vi "Add Project.vi"(6 "Tasks Active?":bool[](array[boolean]), 7 "Add Default Tasks (T)":bool=TRUE, 8 "error in (no error)":errorcluster, 9 "Tasks":string[](array[string]), 10 "Project Name":string, 11 "Projects in":refnum<class "Projects.lvclass">) -> (0 "error out":errorcluster, 3 "Projects out":refnum<class "Projects.lvclass">)   [LabVIEW 2020, in "Projects.lvclass"]
doc: "Adds or updates a project with tasks and sets the active markers all to TRUE in the Project Map in the class data. It defaults to adding the tasks from the default task list as part of the tasks. Nothing will be added if the Project name is empty.\n\n03/2025 Erich Schlieper"
uses:
  Projects.lvclass
  Projects.lvclass/Projects.ctl
  Controls/Project Info.ctl
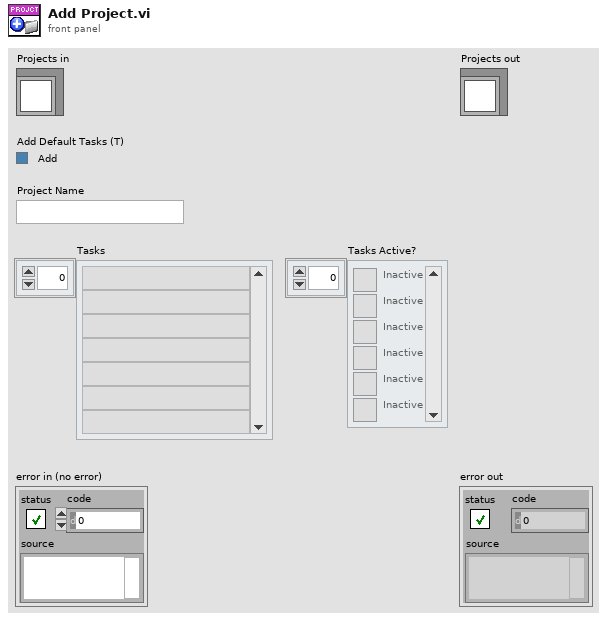
[diagram p1: front panel]
types:
  T1 = typedef "Project Info.ctl" = cluster{"Project Active?":bool, "Tasks":set{string}, "Task Active":map{string, bool}}
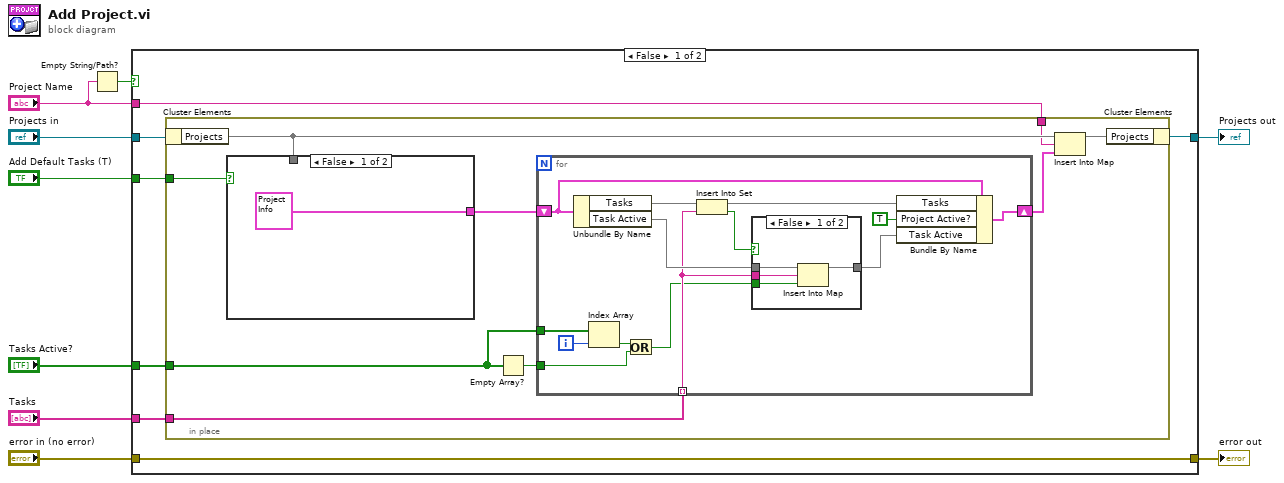
[diagram p0: block diagram]
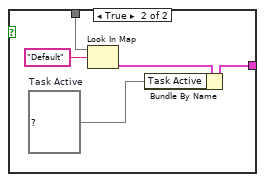
[diagram p3: hidden frame]
diagram:
  n1 = Empty String/Path?(string/path="Project Name") -> (empty?=w2:bool)
  n2 = case shown="False" w2 {
    tunnel: [w15 w52] -> w8
    tunnel: [w14 w51] -> w6
    tunnel: "Projects in" -> [w16 w51]
    tunnel: "Tasks" -> [w11 _]
    tunnel: "Add Default Tasks (T)" -> [w13 _]
    tunnel: "Project Name" -> [w12 _]
    tunnel: "error in (no error)" -> [w15 w52]
    tunnel: "Tasks Active?" -> [w10 _]
    frame False {
      n3 = in-place {
        in-place-border: w13 -> [w23]
        in-place-border: w12 -> [w21]
        in-place-border: w11 -> [w20]
        in-place-border: w10 -> [w18]
        n4 = in-place-cluster #1(w16) -> ("Projects"=w24:map{string, T1})
        n5 = case shown="False" w23 {
          tunnel: w24 -> [_ w50]
          tunnel: [T1 {"Project Active?"=FALSE, "Tasks"={}, "Task Active"={}} ("Project Info") w47] -> w22
          frame False {
          }
          frame True {
            w46 = map{string, bool} {}  # Task Active
            n6 = Look In Map(map=w50, key="Default") -> (value=w48:T1)  [unwired: 1 in, 1 out]
            n7 = Bundle By Name(cluster=w48, "Task Active"=w46) -> (w47:T1)
          }
        }
        n8 = Empty Array?(array=w18) -> (empty?=w17:bool)
        n9 = for {
          shift-right: [w37] -> w19
          shift-left: w22 -> [w36]
          tunnel: w20 -> [w31] mode=indexing
          tunnel: w18 -> [w29]
          tunnel: w17 -> [w27]
          i -> [w30]
          n10 = Unbundle By Name(w36) -> ("Tasks"=w38:set{string}, "Task Active"=w33:map{string, bool})
          n11 = Index Array(array=w29, index=w30) -> (element=w28:bool)
          n12 = Or(x=w28, y=w27) -> (x .or. y?=w26:bool)
          n13 = Insert Into Set(10:w31, 11:w38) -> (2:w34:bool, 3:w39:set{string})
          n14 = case shown="False" w34 {
            tunnel: w33 -> [w43 w44]
            tunnel: [w42 w44] -> w32
            tunnel: w31 -> [w41 _]
            tunnel: w26 -> [w40 _]
            frame False {
              n15 = Insert Into Map(map in=w43, key=w41, value=w40) -> (map out=w42:map{string, bool})  [unwired: 2 out]
            }
            frame True {
            }
          }
          n16 = Bundle By Name(cluster=w36, "Tasks"=w39, "Project Active?"=TRUE, "Task Active"=w32) -> (w37:T1)
        }
        n17 = Insert Into Map(map in=w24, key=w21, value=w19) -> (map out=w25:map{string, T1})  [unwired: 2 out]
        n18 = in-place-cluster #1("Projects"=w25) -> (w14:refnum<class "Projects.lvclass">)
      }
    }
    frame True {
    }
  }
  "error out" <- w8
  "Projects out" <- w6
